vi "Read XNET Frame.vi"(8 "error in (no error)":errorcluster, 11 "XNET Data in":refnum<class "XNET Data.lvclass">) -> (0 "error out":errorcluster, 2 "XNET Frame":refnum<k21>, 3 "XNET Data out":refnum<class "XNET Data.lvclass">)   [LabVIEW 2021, in "BS120x Driver.lvlib" / "Data Classes.lvlib" / "XNET Data.lvclass"]
uses:
  XNET Data.lvclass
  XNET Data.lvclass/XNET Data.ctl
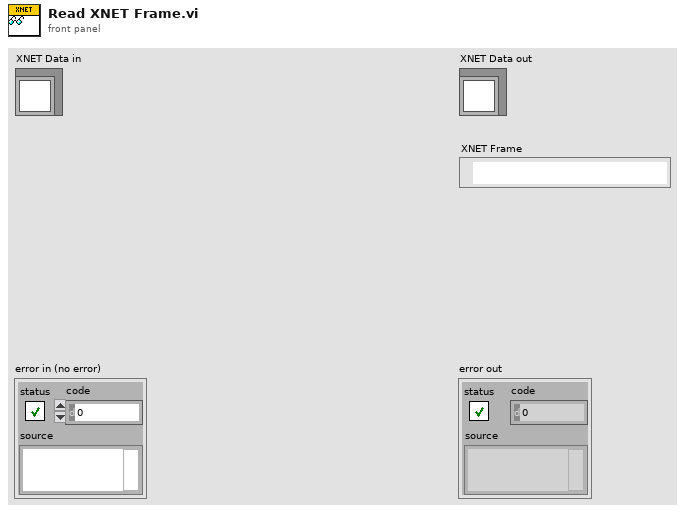
[diagram p1: front panel]
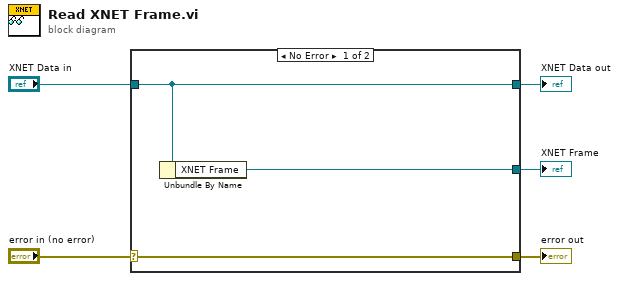
[diagram p0: block diagram]
diagram:
  n1 = case shown="No Error" "error in (no error)" {
    selector: "error in (no error)" -> [w8 w9]
    tunnel: [w8 w9] -> w4
    tunnel: [w7 w10] -> w2
    tunnel: "XNET Data in" -> [w7 w10]
    tunnel: [w6 _] -> w1
    frame No Error {
      n2 = Unbundle By Name(w7) -> ("XNET Frame"=w6:refnum<k21>)
    }
    frame Error {
    }
  }
  "error out" <- w4
  "XNET Data out" <- w2
  "XNET Frame" <- w1
